vi "Init.vi"(11 "Options":T1[](array[typedef])) -> (0 "error out":errorcluster, 2 "Option Set out":refnum<class "Option Set.lvclass">, 3 "CLI out":refnum<class "CLI.lvclass">)   [LabVIEW 2016, in "Script.lvlib"]
uses:
  Script.lvlib
  <vilib>/Wiresmith Technology/G CLI/Argument Parser/Option Set Class/Option Set.lvclass
  <vilib>/Wiresmith Technology/G CLI/Argument Parser/Option Class/Option Configuration.ctl
  <vilib>/Wiresmith Technology/G CLI/Argument Parser/Option Class/Argument Type.ctl
  <vilib>/Wiresmith Technology/G CLI/CLI Class/CLI.lvclass
  <vilib>/Wiresmith Technology/G CLI/Argument Parser/Option Class/Option.lvclass
panel:
  in  "error in (no error)":errorcluster
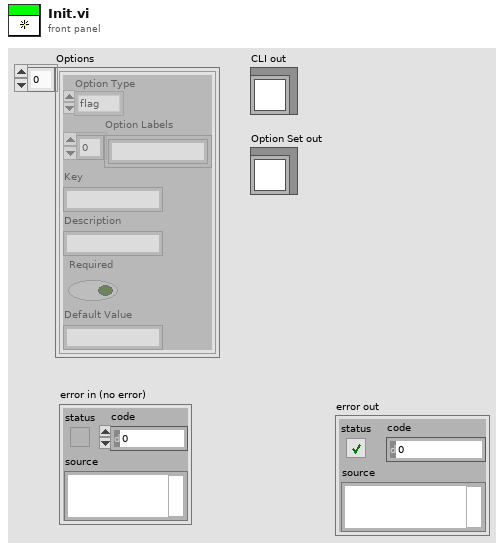
[diagram p1: front panel]
types:
  T1 = typedef "Option Parser.lvlib/Option.lvclass/Option Configuration.ctl" = cluster{"Option Type":T2, "Option Labels":string[], "Key":string, "Description":string, "Required":bool, "Default Value":string}
  T2 = typedef "Option Parser.lvlib/Option.lvclass/Argument Type.ctl" = enum16{"flag", "value"}
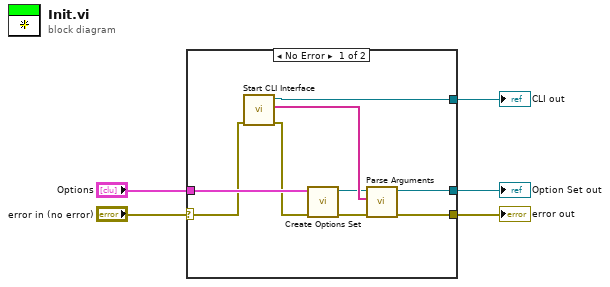
[diagram p0: block diagram]
diagram:
  n1 = case shown="No Error" "error in (no error)" {
    selector: "error in (no error)" -> [w6 w15]
    tunnel: [w14 _] -> w5
    tunnel: [w13 w15] -> w4
    tunnel: "Options" -> [w12 _]
    tunnel: [w7 _] -> w2
    frame No Error {
      n2 = call <vilib>:"Start CLI Interface.vi"("error in (no error)"=w6) -> ("error out"=w11:errorcluster, "Custom Parameters"=w10:string[], "CLI out"=w7:refnum<class "CLI.lvclass">)  [unwired: 7 in, 1 out]
      n3 = call <vilib>:"Create Options Set.vi"("error in (no error)"=w11, "Options"=w12) -> ("error out"=w9:errorcluster, "Option Set out"=w8:refnum<class "Option Set.lvclass">)  [unwired: 8 in]
      n4 = call <vilib>:"Parse Arguments.vi"("error in (no error)"=w9, "Arguments"=w10, "Option Set in"=w8) -> ("error out"=w13:errorcluster, "Option Set out"=w14:refnum<class "Option Set.lvclass">)  [unwired: 5 in, 2 out]
    }
    frame Error {
    }
  }
  "Option Set out" <- w5
  "error out" <- w4
  "CLI out" <- w2
